vi "wait_for_OPC.vi"(5 "Timeout in (0 = OPC timeout)":u32, 7 "Attribute":T1={"Identifier"="", "Descriptive name"="", "Data Type"=enum."Integer 32", "Command"="", "Access"=2, "Range Table"="", "Read Callback"="", "Write Callback"="", "Range Callback"="", "Check Callback"="", "Rngtable Callback"="", "Coerce Callback"="", "Supported Models"="", "Instrument Options"="", "Repeated Capabilities"="", "Check Status Callback"="", "Index"=0, "Flag: OPC Wait"=FALSE, "Flag: Dont check status"=FALSE, "Flag: Cache Only"=FALSE} {"Access" items=["Read Only", "Write Only", "Read/Write"]}, 8 "error in":errorcluster, 10 "STB Bits filter (No Filter - 0xFF)":u16(ring)=255 format="0x%02x" items=["No Filter"=255, "ERR+MAV+ESB(OPC)"=52, "ERR+MAV"=20, "ERR+ESB(OPC)"=36], 11 "VISA resource name":refnum<visa-resource-name>) -> (0 "error out":errorcluster, 3 "VISA resource name out":refnum<visa-resource-name>)   [LabVIEW 2014, in "rszvl_rsidr_core.lvlib"]
uses:
  rszvl_rsidr_core.lvlib
  type_Attribute.ctl
  type_Attribute_Data_Type.ctl
  type_Error_Codes.ctl
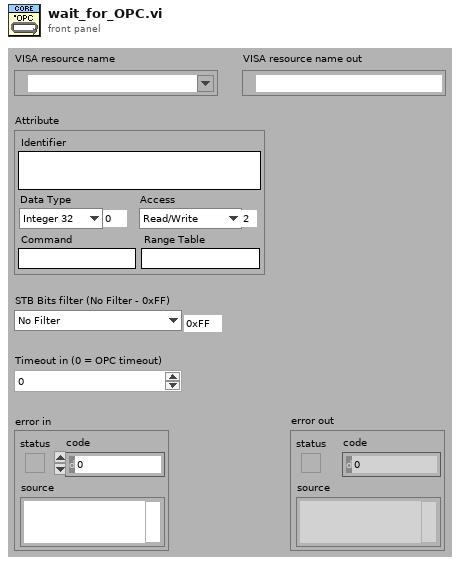
[diagram p1: front panel]
types:
  T1 = typedef "rszvl_rsidr_core.lvlib/type_Attribute.ctl" = cluster{"Identifier":string, "Descriptive name":string, "Data Type":T2, "Command":string, "Access":u16, "Range Table":string, "Read Callback":string, "Write Callback":string, "Range Callback":string, "Check Callback":string, "Rngtable Callback":string, "Coerce Callback":string, "Supported Models":string, "Instrument Options":string, "Repeated Capabilities":string, "Check Status Callback":string, "Index":i32, "Flag: OPC Wait":bool, "Flag: Dont check status":bool, "Flag: Cache Only":bool}
  T2 = typedef "rszvl_rsidr_core.lvlib/type_Attribute_Data_Type.ctl" = enum16{"Integer 32", "Double", "String", "Boolean", "None", "Integer 64"}
  T3 = enum16{"Check error", "Don't check error", "Check error from Session"}
  T4 = typedef "rszvl_rsidr_core.lvlib/type_Error_Codes.ctl" = enum16{"No_error", "VISA_err_ResourceNotFound", "VISA_err_Timeout", "VISA_warn_MoreDataAvailable", "RS_err_MissingCallback", "RS_err_InvalidAttribute", "RS_err_InvalidValue", "RS_err_UnknownResource", "RS_err_AlreadyInitialized", "RS_err_InstrumentStatus", "RS_err_BadRepCapName", "RS_err_TypesMismatch", "RS_err_ValueNotSupported", "RS_err_InvalidRngTable", "RS_err_IDqueryFail", "RS_err_UnexpResponse", "VISA_warn_ConfigNotLoaded", "RS_err_AttributeNotReadable", "RS_err_AttributeNotWritable", "RS_err_InstrumentType", "RS_err_InstrumentOption", "VISA_err_InvalidSize", "RS_err_ReliabilityIndicator", "VISA_warn_UnknownStatus", "VISA_warn_TermCharRead", "VISA_err_IO_error"}
  T5 = typedef "rszvl_rsidr_core.lvlib/type_Session_Data.ctl" = cluster{"Instr type":string, "Instr type for err. msg.":string, "Installed Options":string[], "OPC Timeout":i32, "Query Instrument Status":bool, "Check Range":bool, "Check Options":bool, "Add LF to Write":bool, "Simulate":bool, "Logging":bool, "Logging params":variant, "Interface Type":enum16{"Unknown", "GPIB", "VXI", "GPIB_VXI", "ASRL", "PXI", "TCPIP", "USB", "SOCKET"}, "Fast Sweep":i32, "AdditionalFlags":i32, "WaitBeforeWrite":i32, "WaitBeforeRead":i32, "BinDataChunkSize":i64}
  T6 = enum16{"Unknown", "GPIB", "VXI", "GPIB_VXI", "ASRL", "PXI", "TCPIP", "USB", "SOCKET"}
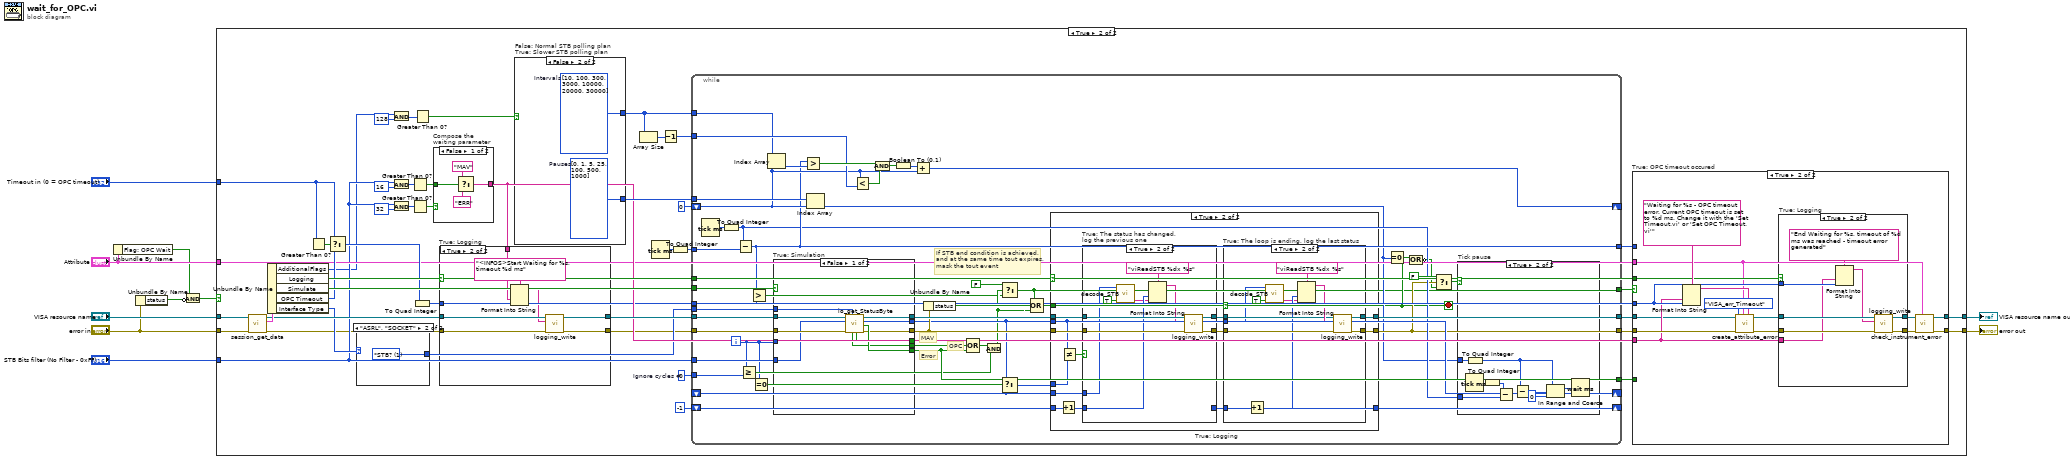
[diagram p0: block diagram]
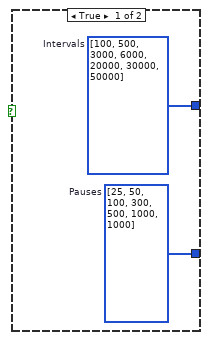
[diagram p3: hidden frame]
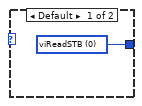
[diagram p4: hidden frame]
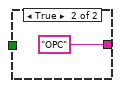
[diagram p5: hidden frame]
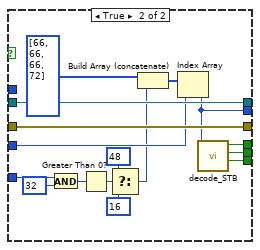
[diagram p8: hidden frame]
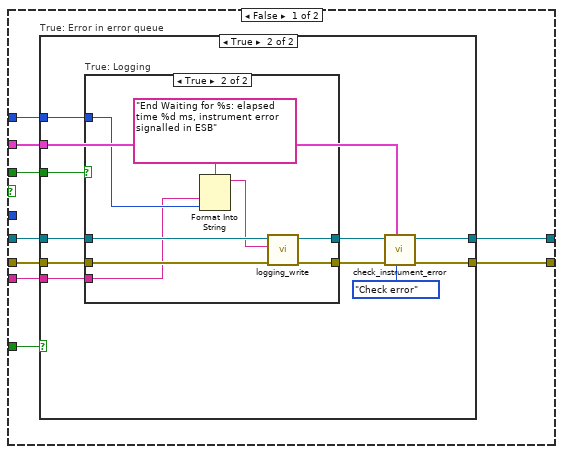
[diagram p12: hidden frame]
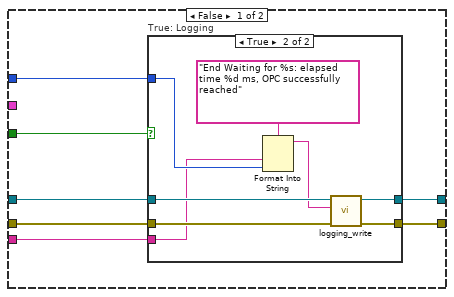
[diagram p13: hidden frame]
diagram:
  n1 = Unbundle By Name("Attribute") -> ("Flag: OPC Wait"=w2:bool)
  n2 = Unbundle By Name("error in") -> ("status"=w3:bool)
  n3 = Compound Arithmetic op=AND(w2, invert w3) -> (w1:bool)
  n4 = case shown="True" w1 {
    tunnel: "VISA resource name" -> [w12 w55]
    tunnel: "error in" -> [w11 w54]
    tunnel: [w12 w27] -> w9
    tunnel: [w11 w26] -> w10
    tunnel: "Timeout in (0 = OPC timeout)" -> [_ w29]
    tunnel: "Attribute" -> [_ w25]
    tunnel: "STB Bits filter (No Filter - 0xFF)" -> [_ w20]
    frame False {
    }
    frame True {
      w21 = 0  # Ignore cycles #
      n5 = call "session_get_data.vi"("error in"=w54, "VISA resource name"=w55) -> ("error out"=w18:errorcluster, "Session User Data out"=w53:T5, "VISA resource name out"=w52:refnum<visa-resource-name>)  [unwired: 7 in]
      n6 = Unbundle By Name(w53) -> ("AdditionalFlags"=w16:i32, "Logging"=w40:bool, "Simulate"=w41:bool, "OPC Timeout"=w32:i32, "Interface Type"=w23:T6)
      n7 = Greater Than 0?(x=w29) -> (x > 0?=w30:bool)
      n8 = Select(t=w29, s=w30, f=w32) -> (s? t:f=w28:u32)
      n9 = case shown="\"ASRL\", \"SOCKET\"" w23 {
        tunnel: [w60 w61] -> w22
        frame Default {
          w60 = u16 0 items=["viReadSTB", "*STB?"] ("Method (viReadSTB)")
        }
        frame "ASRL", "SOCKET" {
          w61 = u16 1 items=["viReadSTB", "*STB?"] ("Method (viReadSTB)")
        }
      }
      n10 = And(x=w16, y=128) -> (x .and. y?=w14:i32)
      n11 = And(x=w20, y=u16 16) -> (x .and. y?=w39:u16)
      n12 = And(x=w20, y=u16 32) -> (x .and. y?=w36:u16)
      n13 = Greater Than 0?(x=w39) -> (x > 0?=w35:bool)
      n14 = Greater Than 0?(x=w36) -> (x > 0?=w34:bool)
      n15 = To Quad Integer(1:w28) -> (0:w31:i64)
      n16 = Greater Than 0?(x=w14) -> (x > 0?=w13:bool)
      n17 = case "Compose the\nwaiting parameter" shown="False" w34 {
        tunnel: w35 -> [w62 _]
        tunnel: [w65 "OPC"] -> w33
        frame False {
          n18 = Select(t="MAV", s=w62, f="ERR") -> (s? t:f=w65:string)
        }
        frame True {
        }
      }
      n19 = case "True: Logging" shown="True" w40 {
        tunnel: [w68 w76] -> _
        tunnel: [w67 w75] -> _
        tunnel: w18 -> [w68 w69]
        tunnel: w52 -> [w67 w70]
        tunnel: w33 -> [_ w72]
        tunnel: w31 -> [_ w71]
        frame False {
        }
        frame True {
          n20 = Format Into String(format string="<INFOS>Start Waiting for %s, timeout %d ms", w72, w71) -> (resulting string=w74:string)  [unwired: 2 in, 1 out]
          n21 = call "logging_write.vi"("error in"=w69, "String to write"=w74, "VISA resource name"=w70) -> ("error out"=w76:errorcluster, "VISA resource name out"=w75:refnum<visa-resource-name>)  [unwired: 7 in]
        }
      }
      n22 = case "False: Normal STB polling plan\nTrue: Slower STB polling plan" shown="False" w13 {
        tunnel: [w57 w58] -> w49
        tunnel: [w56 w59] -> w48
        frame True {
          w57 = u32[] [25, 50, 100, 300, 500, 1000, 1000]  # Pauses
          w56 = i32[] [100, 500, 3000, 6000, 20000, 30000, 50000]  # Intervals
        }
        frame False {
          w58 = u32[] [0, 1, 5, 25, 100, 500, 1000]  # Pauses
          w59 = i32[] [10, 100, 300, 3000, 10000, 20000, 30000]  # Intervals
        }
      }
      n23 = Array Size(array=w48) -> (size(s)=w46:i32)
      n24 = Tick Count (ms)() -> (millisecond timer value=w51:u32)
      n25 = Decrement(x=w46) -> (x-1=w45:i32)
      n26 = To Quad Integer(1:w51) -> (0:w19:i64)
      n27 = while {
        tunnel: [w79] -> w24
        tunnel: w19 -> [w125]
        tunnel: w31 -> [w85]
        tunnel: [w106] -> w44
        tunnel: w52 -> [w112]
        tunnel: [w111] -> w50
        shift-right: [w117] -> _
        shift-left: 0 -> [w113]
        tunnel: w48 -> [w116]
        tunnel: w49 -> [w118]
        tunnel: w45 -> [w119]
        tunnel: [w93] -> w43
        shift-right: [w100] -> _
        shift-left: _ -> [w99]
        tunnel: w40 -> [w98]
        shift-right: [w104] -> _
        shift-left: -1 -> [w105]
        tunnel: w41 -> [w102]
        tunnel: w21 -> [w101]
        tunnel: w20 -> [w96]
        tunnel: w22 -> [w95]
        tunnel: w18 -> [w87]
        tunnel: [w86] -> w17
        i -> [w94]
        stop <- w82 stop-if-true
        # "If STB end condition is achieved,\nand at the same time tout expires,\nmask the tout event"
        # "OPC"
        # "Error"
        # "MAV"
        n28 = Tick Count (ms)() -> (millisecond timer value=w91:u32)
        n29 = To Quad Integer(1:w91) -> (0:w88:i64)
        n30 = Subtract(x=w88, y=w125) -> (x-y=w93:i64)
        n31 = Greater Or Equal?(x=w94, y=w101) -> (x >= y?=w110:bool)
        n32 = Greater?(x=w93, y=w85) -> (0:w78:bool)
        n33 = Equal To 0?(x=w94) -> (x = 0?=w92:bool)
        n34 = Index Array(array=w116, index=w113) -> (element=w120:i32)
        n35 = case "True: Simulation" shown="False" w102 {
          tunnel: w87 -> [w144 w159]
          tunnel: w112 -> [w143 w160]
          tunnel: [w142 w155] -> w111
          tunnel: [w141 w157] -> w109
          tunnel: [w140 w156] -> w108
          tunnel: [w139 w160] -> w107
          tunnel: [w138 w154] -> w100
          tunnel: [w137 w159] -> w103
          tunnel: w94 -> [_ w158]
          tunnel: w96 -> [w136 w151]
          tunnel: w95 -> [w135 _]
          frame False {
            n36 = call "io_get_StatusByte.vi"("Method (viReadSTB)"=w135, "error in"=w144, "Bits filter (None - 0xFF)"=w136, "VISA resource name"=w143) -> ("error out"=w137:errorcluster, "Error"=w142:bool, "STB returned"=w138:u16, "VISA resource name out"=w139:refnum<visa-resource-name>, "MAV"=w140:bool, "OPC (ESB)"=w141:bool)  [unwired: 2 in]
          }
          frame True {
            n37 = And(x=w151, y=u16 32) -> (x .and. y?=w149:u16)
            n38 = Greater Than 0?(x=w149) -> (x > 0?=w148:bool)
            n39 = Select(t=u16 48, s=w148, f=u16 16) -> (s? t:f=w145:u16)
            n40 = Build Array (concatenate)(u16[] [66, 66, 66, 72], w145) -> (w152:u16[])
            n41 = Index Array(array=w152, index=w158) -> (element=w154:u16)
            n42 = call "decode_STB.vi"("STB in"=w154) -> ("Error"=w155:bool, "OPC (ESB)"=w157:bool, "MAV"=w156:bool)  [unwired: 7 in, 1 out]
          }
        }
        n43 = Greater?(x=w93, y=w120) -> (0:w124:bool)
        n44 = Index Array(array=w118, index=w113) -> (element=w84:u32)
        n45 = Less?(x=w113, y=w119) -> (x < y?=w122:bool)
        n46 = Compound Arithmetic op=AND(w124, w122) -> (w123:bool)
        n47 = Boolean To (0,1)(Boolean=w123) -> (0, 1=w121:i16)
        n48 = Add(x=w121, y=w113) -> (x+y=w117:i32)
        n49 = Unbundle By Name(w103) -> ("status"=w115:bool)
        n50 = Compound Arithmetic op=OR(w108, w109, w111) -> (w114:bool)
        n51 = Compound Arithmetic op=AND(w114, w110) -> (w80:bool)
        n52 = Select(t=w100, s=w92, f=w99) -> (s? t:f=w97:u16)
        n53 = Select(t=FALSE, s=w80, f=w78) -> (s? t:f=w79:bool)
        n54 = Compound Arithmetic op=OR(w79, w115, w80) -> (w82:bool)
        n55 = case "True: Logging" shown="True" w98 {
          tunnel: [w163 w170] -> w86
          tunnel: [w162 w169] -> w106
          tunnel: w103 -> [w163 w177]
          tunnel: w107 -> [w162 w176]
          tunnel: w105 -> [w161 w166]
          tunnel: [w161 w164] -> w104
          tunnel: w100 -> [_ w167]
          tunnel: w99 -> [_ w175]
          tunnel: w97 -> [_ w174]
          tunnel: w82 -> [_ w168]
          frame False {
          }
          frame True {
            n56 = Increment(x=w166) -> (x+1=w165:i32)
            n57 = Not Equal?(x=w167, y=w174) -> (x != y?=w173:bool)
            n58 = case "True: The status has changed,\nlog the previous one" shown="True" w173 {
              tunnel: w177 -> [w192 w203]
              tunnel: w176 -> [w193 w202]
              tunnel: [w192 w201] -> w172
              tunnel: [w193 w200] -> w171
              tunnel: w165 -> [w191 w195]
              tunnel: w175 -> [_ w199]
              tunnel: [w191 _] -> w164
              frame False {
              }
              frame True {
                n59 = call "decode_STB.vi"("Compose Summary String  (F)"=TRUE, "STB in"=w199) -> ("Summary string"=w194:string)  [unwired: 6 in, 3 out]
                n60 = Format Into String(format string="viReadSTB %dx %s" ("String to write"), w195, w194) -> (resulting string=w196:string)  [unwired: 2 in, 1 out]
                n61 = call "logging_write.vi"("error in"=w203, "String to write"=w196, "VISA resource name"=w202) -> ("error out"=w201:errorcluster, "VISA resource name out"=w200:refnum<visa-resource-name>)  [unwired: 7 in]
              }
            }
            n62 = case "True: The loop is ending, log the last status" shown="True" w168 {
              tunnel: w172 -> [w178 w187]
              tunnel: w171 -> [w179 w186]
              tunnel: [w178 w185] -> w170
              tunnel: [w179 w184] -> w169
              tunnel: w167 -> [_ w183]
              tunnel: w164 -> [_ w182]
              frame False {
              }
              frame True {
                n63 = Increment(x=w182) -> (x+1=w181:i32)
                n64 = call "decode_STB.vi"("Compose Summary String  (F)"=TRUE, "STB in"=w183) -> ("Summary string"=w180:string)  [unwired: 6 in, 3 out]
                n65 = Format Into String(format string="viReadSTB %dx %s" ("String to write"), w181, w180) -> (resulting string=w188:string)  [unwired: 2 in, 1 out]
                n66 = call "logging_write.vi"("error in"=w187, "String to write"=w188, "VISA resource name"=w186) -> ("error out"=w185:errorcluster, "VISA resource name out"=w184:refnum<visa-resource-name>)  [unwired: 7 in]
              }
            }
          }
        }
        n67 = Equal To 0?(x=w84) -> (x = 0?=w83:bool)
        n68 = Compound Arithmetic op=OR(w83, w82) -> (invert w81:bool)
        n69 = Select(t=FALSE, s=w86, f=w81) -> (s? t:f=w90:bool)
        n70 = case "Tick pause" shown="True" w90 {
          tunnel: w88 -> [_ w133]
          tunnel: w84 -> [_ w130]
          frame False {
          }
          frame True {
            n71 = Tick Count (ms)() -> (millisecond timer value=w134:u32)
            n72 = To Quad Integer(1:w130) -> (0:w126:i64)
            n73 = To Quad Integer(1:w134) -> (0:w129:i64)
            n74 = Subtract(x=w129, y=w133) -> (x-y=w128:i64)
            n75 = Subtract(x=w126, y=w128) -> (x-y=w127:i64)
            n76 = In Range and Coerce(upper limit=w126, x=w127, lower limit=i64 0) -> (coerced(x)=w131:i64)  [unwired: 1 out]
            n77 = Wait (ms)(milliseconds to wait=w131) -> ()  [unwired: 1 out]
          }
        }
      }
      n78 = case "True: OPC timeout occured" shown="True" w24 {
        tunnel: w44 -> [w209 w258]
        tunnel: w17 -> [w211 w265]
        tunnel: [w210 w252] -> w26
        tunnel: [w208 w251] -> w27
        tunnel: w50 -> [w212 _]
        tunnel: w25 -> [w207 w253]
        tunnel: w31 -> [_ w261]
        tunnel: w40 -> [w205 w260]
        tunnel: w43 -> [w206 _]
        tunnel: w33 -> [w204 w259]
        frame False {
          n79 = case "True: Error in error queue" shown="True" w212 {
            tunnel: w211 -> [w218 w235]
            tunnel: [w216 w240] -> w210
            tunnel: w209 -> [w219 w236]
            tunnel: [w217 w239] -> w208
            tunnel: w207 -> [_ w238]
            tunnel: w206 -> [w215 w234]
            tunnel: w205 -> [w214 w233]
            tunnel: w204 -> [w213 w230]
            frame False {
              n80 = case "True: Logging" shown="True" w214 {
                tunnel: [w221 w227] -> w216
                tunnel: [w220 w226] -> w217
                tunnel: w218 -> [w221 w229]
                tunnel: w219 -> [w220 w228]
                tunnel: w215 -> [_ w223]
                tunnel: w213 -> [_ w222]
                frame False {
                }
                frame True {
                  n81 = Format Into String(format string="End Waiting for %s: elapsed time %d ms, OPC successfully reached", w222, w223) -> (resulting string=w225:string)  [unwired: 2 in, 1 out]
                  n82 = call "logging_write.vi"("error in"=w229, "String to write"=w225, "VISA resource name"=w228) -> ("error out"=w227:errorcluster, "VISA resource name out"=w226:refnum<visa-resource-name>)  [unwired: 7 in]
                }
              }
            }
            frame True {
              n83 = case "True: Logging" shown="True" w233 {
                tunnel: [w242 w248] -> w231
                tunnel: [w241 w247] -> w232
                tunnel: w235 -> [w242 w250]
                tunnel: w236 -> [w241 w249]
                tunnel: w234 -> [_ w244]
                tunnel: w230 -> [_ w243]
                frame False {
                }
                frame True {
                  n84 = Format Into String(format string="End Waiting for %s: elapsed time %d ms, instrument error signalled in ESB", w243, w244) -> (resulting string=w246:string)  [unwired: 2 in, 1 out]
                  n85 = call "logging_write.vi"("error in"=w250, "String to write"=w246, "VISA resource name"=w249) -> ("error out"=w248:errorcluster, "VISA resource name out"=w247:refnum<visa-resource-name>)  [unwired: 7 in]
                }
              }
              n86 = call "check_instrument_error.vi"("Mode (Check error from Session)"=T3."Check error", "Attribute"=w238, "error in"=w231, "VISA resource name"=w232) -> ("error out"=w240:errorcluster, "VISA resource name out"=w239:refnum<visa-resource-name>)  [unwired: 6 in]
            }
          }
        }
        frame True {
          n87 = Format Into String(format string="Waiting for %s - OPC timeout error. Current OPC timeout is set to %d ms. Change it with the 'Set Timeout.vi' or 'Set OPC Timeout.vi'", w259, w261) -> (resulting string=w263:string)  [unwired: 2 in, 1 out]
          n88 = call "create_attribute_error.vi"("Error Elaboration (\"\")"=w263, "Attribute"=w253, "error in"=w265, "Error Enum in"=type_Error_Codes."VISA_err_Timeout" ("Error Enum in (from err to recompose)"), "VISA resource name"=w258) -> ("error out"=w262:errorcluster, "VISA resource name out"=w257:refnum<visa-resource-name>)  [unwired: 5 in]
          n89 = case "True: Logging" shown="True" w260 {
            tunnel: [w267 w273] -> w255
            tunnel: [w266 w272] -> w254
            tunnel: w262 -> [w267 w275]
            tunnel: w257 -> [w266 w274]
            tunnel: w261 -> [_ w269]
            tunnel: w259 -> [_ w268]
            frame False {
            }
            frame True {
              n90 = Format Into String(format string="End Waiting for %s, timeout of %d ms was reached - timeout error generated", w268, w269) -> (resulting string=w271:string)  [unwired: 2 in, 1 out]
              n91 = call "logging_write.vi"("error in"=w275, "String to write"=w271, "VISA resource name"=w274) -> ("error out"=w273:errorcluster, "VISA resource name out"=w272:refnum<visa-resource-name>)  [unwired: 7 in]
            }
          }
          n92 = call "check_instrument_error.vi"("Attribute"=w253, "error in"=w255, "VISA resource name"=w254) -> ("error out"=w252:errorcluster, "VISA resource name out"=w251:refnum<visa-resource-name>)  [unwired: 7 in]
        }
      }
    }
  }
  "VISA resource name out" <- w9
  "error out" <- w10
